vi "LightsMath.vi"(10 "Shooter RPM":dbl) -> (2 "Light Timing":dbl)   [LabVIEW 2011]
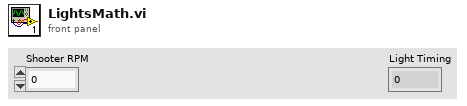
[diagram p1: front panel]
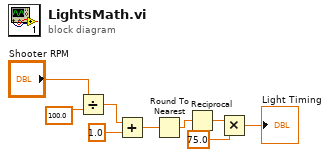
[diagram p0: block diagram]
diagram:
  n1 = Divide(x="Shooter RPM", y=100.0) -> (x/y=w8:dbl)
  n2 = Add(x=w8, y=1.0) -> (x+y=w6:dbl)
  n3 = Round To Nearest(number=w6) -> (nearest integer value=w5:dbl)
  n4 = Reciprocal(x=w5) -> (1/x=w4:dbl)
  n5 = Multiply(x=w4, y=75.0) -> (x*y=→"Light Timing":dbl)
